vi "TEST_bench_FXP_A_times_x_iterate_32bit.vi"(6 "NS":u8=9) -> ()   [LabVIEW 2017]
uses:
  fpga_subVIs_ssxy/fixed-point-ss/typeDefs/UT_matrix_data.ctl
  fpga_subVIs_ssxy/fixed-point-ss/typeDefs/Bz_vec_scalar.ctl
  fpga_subVIs_ssxy/fixed-point-ss/typeDefs/Lz_vec_scalar.ctl
  fpga_subVIs_ssxy/fixed-point-ss/typeDefs/Kz_vec_scalar.ctl
  fpga_subVIs_ssxy/fixed-point-ss/typeDefs/Nx_vec_scalar.ctl
  fpga_subVIs_ssxy/fixed-point-ss/typeDefs/Az_vec_scalar.ctl
  fpga_subVIs_ssxy/fixed-point-ss/typeDefs/x_vec_scalar.ctl
  fpga_subVIs_ssxy/fixed-point-ss/typeDefs/Cz_vec_scalar.ctl
  fpga_subVIs_ssxy/fixed-point-ss/typeDefs/x_vec_bram.ctl
  fpga_subVIs_ssxy/fixed-point-ss/typeDefs/A_as_vec_bram.ctl
  <vilib>/rvi/DataTransferAndStorage/Container/Common/niFpgaContainerExecOnDevCompGetState.vi
  <vilib>/rvi/Emulation/niFpgaEmulationIsFPGAContextNoSignature.vi
  <vilib>/rvi/DataTransferAndStorage/Container/Common/niFpgaContainerGetUniqueNameForEmu.vi
  <vilib>/rvi/Emulation/niFpgaProcessEmulError.vi
  <vilib>/rvi/Emulation/niFpgaSctlEmulationGetInTimedLoop.vi
  <vilib>/rvi/errors/nirviReportUnexpectedCaseInternalError (U32).vi
  <vilib>/rvi/Memory/Memory_Emulation/niFpgaMemoryEmulationCacheClearOnFirstRun.vi
  <vilib>/rvi/Memory/Memory_Emulation/nirvimemoryEmulationManagerCache_MakeExclusive.vi
  <vilib>/rvi/Memory/Memory_Emulation/niFpgaMemoryEmulationValidateCache.vi
  <vilib>/rvi/Memory/Memory_Emulation/nirvimemoryEmulationManagerCache_InsertValue.vi
  <vilib>/Utility/error.llb/Clear Errors.vi
  <vilib>/rvi/Memory/Memory_Emulation/nirvimemoryEmulationManagerCache_ReleaseExclusive.vi
  <vilib>/rvi/Memory/Memory_Emulation/nirvimemoryEmulationManagerCache_GetValue.vi
  <vilib>/rvi/Memory/Memory_Emulation/nirvimemoryEmulationManagerCache_SetValue.vi
  <vilib>/rvi/Emulation/niFpgaSctlEmulationResourceMgr.vi
  <vilib>/rvi/DataTransferAndStorage/Container/XNode/niFpgaContainer.xnode
  <vilib>/rvi/Memory/Memory_Emulation/niFpgaMemoryEmulationRefIn.vi
panel:
  in  "matrix data":T1
  out "xk_1_1":fxp<+/-,32,6>[](array[numeric])
  out "A*x":fxp<+/-,32,13>[](array[numeric])
  in  "NumIter":i32
  out "Y":fxp<+/-,32,6>[](array[numeric])
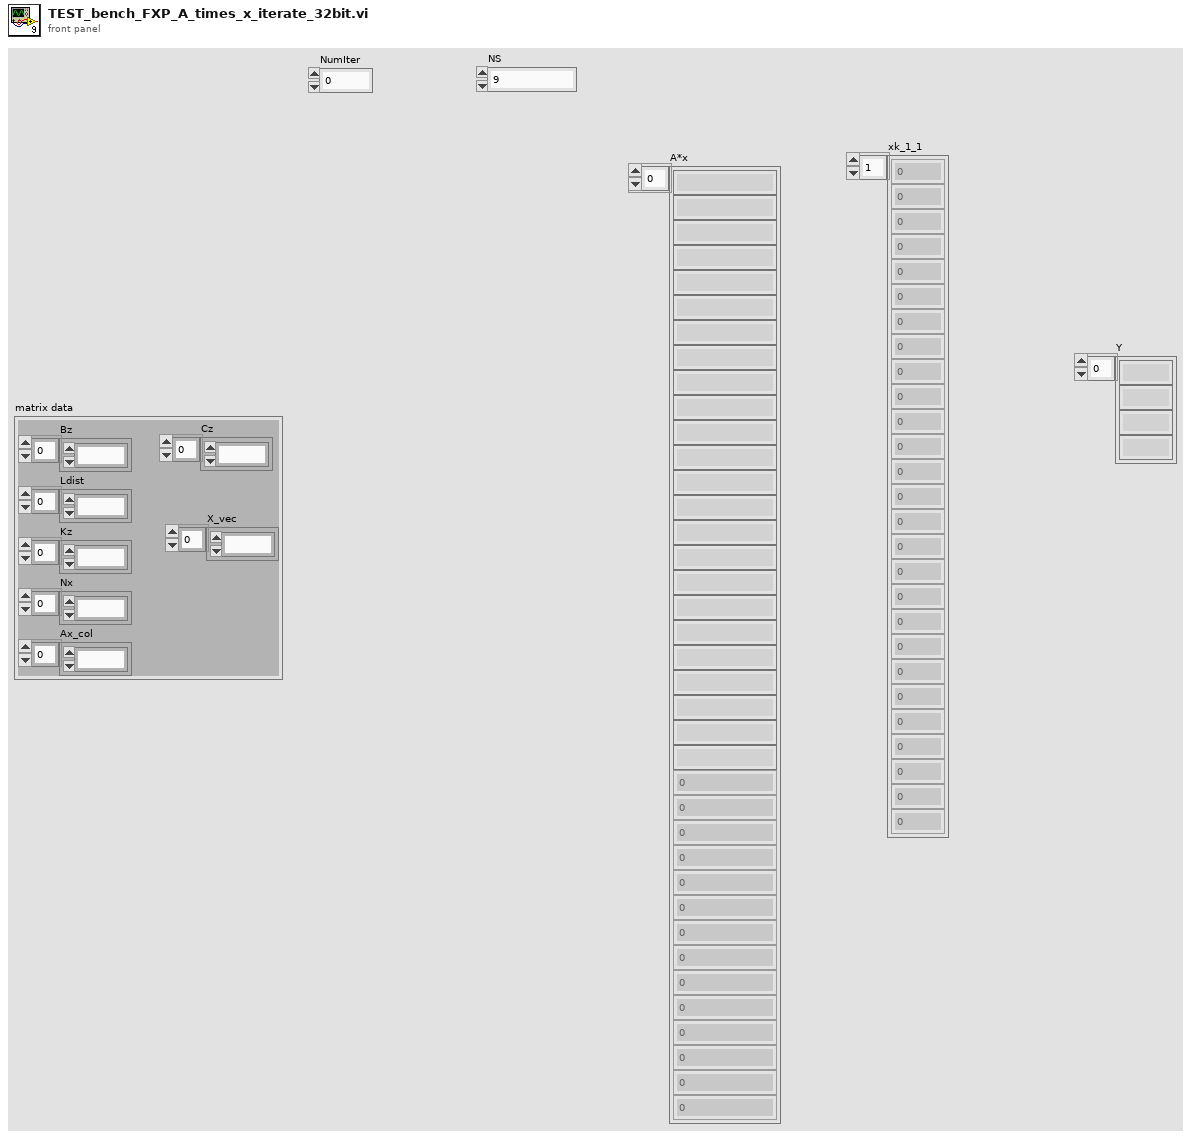
[diagram p1: front panel]
types:
  T1 = typedef "UT_matrix_data.ctl" = cluster{"Bz":T2[], "Ldist":T3[], "Kz":T4[], "Nx":T5[], "Ax_col":T6[], "X_vec":T7[], "Cz":T8[]}
  T2 = typedef "Bz_vec_scalar.ctl" = fxp<+/-,32,3>
  T3 = typedef "Lz_vec_scalar.ctl" = fxp<+/-,32,3>
  T4 = typedef "Kz_vec_scalar.ctl" = fxp<+/-,32,10>
  T5 = typedef "Nx_vec_scalar.ctl" = fxp<+/-,32,2>
  T6 = typedef "Az_vec_scalar.ctl" = fxp<+/-,32,7>
  T7 = typedef "x_vec_scalar.ctl" = fxp<+/-,32,6>
  T8 = typedef "Cz_vec_scalar.ctl" = fxp<+/-,32,4>
  T9 = typedef "x_vec_bram.ctl" = refnum<k21>
  T10 = typedef "A_as_vec_bram.ctl" = refnum<k21>
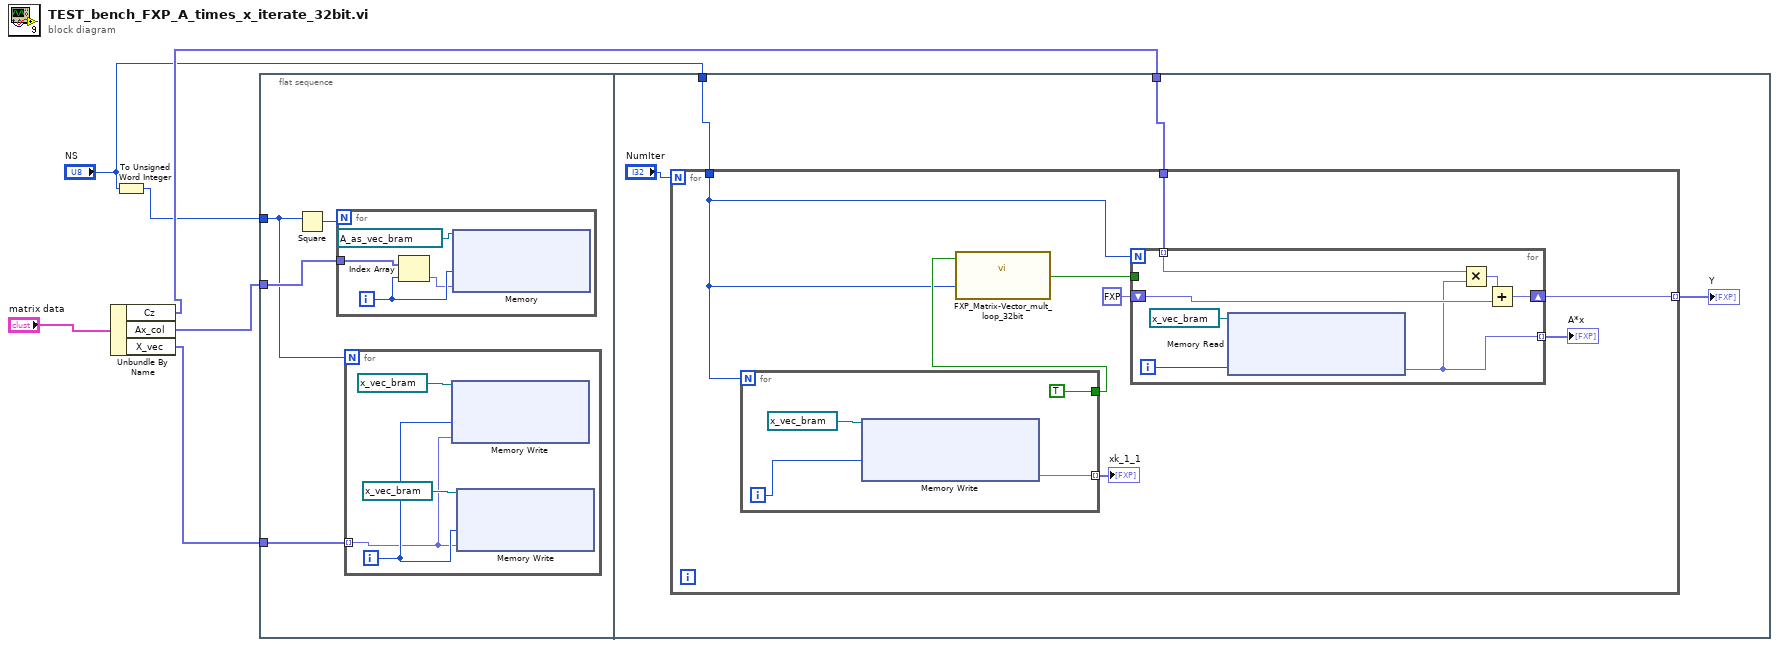
[diagram p0: block diagram]
diagram:
  n1 = Unbundle By Name("matrix data") -> ("Cz"=w4:T8[], "Ax_col"=w6:T6[], "X_vec"=w5:T7[])
  n2 = To Unsigned Word Integer(number="NS") -> (unsigned 16bit integer=w2:u16)
  n3 = flat-sequence {
    tunnel: w2 -> [w7]
    tunnel: w6 -> [w10]
    tunnel: w5 -> [w9]
    tunnel: "NS" -> [w22]
    tunnel: w4 -> [w21]
    frame #0 {
      n4 = Square(x=w7) -> (x^2=w8:u16)
      n5 = for {
        N: w8 -> [_]
        tunnel: w10 -> [w17]
        i -> [w16]
        n6 = Index Array(array=w17, index=w16) -> (element=w15:T6)
        n7 = xnode "Memory"("Address"=w16, "Data"=w15, "Memory In"=T10 "AasCol _FXP") -> ()  [unwired: 1 out]
      }
      n8 = for {
        N: w7 -> [_]
        tunnel: w9 -> [w11] mode=indexing
        i -> [w12]
        n9 = xnode "Memory Write"("Address"=w12, "Data"=w11, "Memory In"=T9 "xk_0_1" ("Memory")) -> ()  [unwired: 1 out]
        n10 = xnode "Memory Write"("Address"=w12, "Data"=w11, "Memory In"=T9 "xk_1_0" ("Memory")) -> ()  [unwired: 1 out]
      }
    }
    frame #1 {
      n11 = for {
        N: "NumIter" -> [_]
        tunnel: w22 -> [w23]
        tunnel: w21 -> [w29]
        tunnel: [w27] -> w20 mode=indexing
        n12 = for {
          N: w23 -> [_]
          tunnel: [w32] -> w26 mode=indexing
          tunnel: [TRUE] -> w25
          i -> [w33]
          n13 = xnode "Memory Write"("Address"=w33, "Memory In"=T9 "xk_0_1" ("Memory")) -> ("Data"=w32:fxp<+/-,32,6>)  [unwired: 1 out]
        }
        "xk_1_1" <- w26
        n14 = call "FXP_Matrix-Vector_mult_loop_32bit.vi"("Ns_1"=w23, "inputValid"=w25) -> ("finished"=w30:bool)  [unwired: 9 in]
        n15 = for {
          N: w23 -> [_]
          tunnel: w30 -> [_]
          tunnel: w29 -> [w41] mode=indexing
          shift-right: [w39] -> w27
          shift-left: fxp<+,32,5> 0.0 -> [w38]
          tunnel: [w35] -> w24 mode=indexing
          i -> [w36]
          n16 = xnode "Memory Read"("Address"=w36, "Memory In"=T9 "xk_1_0" ("Memory")) -> ("Data"=w35:fxp<+/-,32,6>)  [unwired: 1 out]
          n17 = Multiply(x=w41, y=w35) -> (x*y=w40:fxp<+/-,64,10>)
          n18 = Add(x=w40, y=w38) -> (x+y=w39:fxp<+/-,32,5>)
        }
        "A*x" <- w24
      }
      "Y" <- w20
    }
  }
